vi "_emi_New Named Loop Deprecated.vi"(2 "Loop Enabled(T)":bool=TRUE, 7 "Loop Name(\"\")":string, 9 "error in (no error)":errorcluster) -> (6 "Loop ID":u16, 10 "error out":errorcluster)   [LabVIEW 2010]
doc: "Create a new loop vased on name. NOT IMPLEMENTED"
uses:
  _emi_Loop control int action.ctl
  emi_Set Status Loop.vi
  _emi_GFV Loop Running.vi
  _emi_GFV Loop Enable.vi
  _emi_GFV Loop Linking.vi
  _emi_GFV stop a loop so it can reset.vi
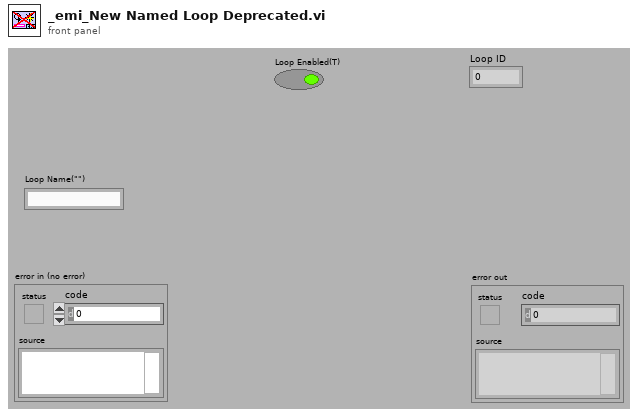
[diagram p1: front panel]
types:
  T1 = typedef "_emi_Loop control int action.ctl" = enum16{"Init index", "Get index", "Set index", "Get Size"}
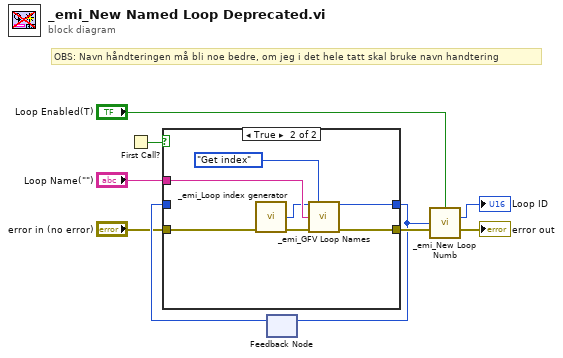
[diagram p0: block diagram]
diagram:
  # "OBS: Navn håndteringen må bli noe bedre, om jeg i det hele tatt skal bruke navn handtering"
  n1 = First Call?() -> (First Call?: T/F=w9:bool)
  n2 = feedback #1() -> (w7:u16)  [unwired: 1 in]
  n3 = case shown="True" w9 {
    tunnel: "Loop Name(\"\")" -> [_ w15]
    tunnel: [w11 w14] -> w3
    tunnel: w7 -> [w11 _]
    tunnel: "error in (no error)" -> [w10 w18]
    tunnel: [w10 w16] -> w5
    frame False {
    }
    frame True {
      n4 = call "_emi_Loop index generator.vi"("error in (no error)"=w18) -> ("Loop ID out"=w12:u16, "error out"=w17:errorcluster)  [unwired: 13 in]
      n5 = call "_emi_GFV Loop Names.vi"("Loop Index/Numb"=w12, "Action(Get Index)"=_emi_Loop_control_int_action."Get index", "Loop Name(\"\")"=w15, "error in (no error)"=w17) -> ("Index out"=w14:u16, "error out"=w16:errorcluster)  [unwired: 8 in, 2 out]
    }
  }
  n6 = feedback-in #1(w3) -> ()
  n7 = call "_emi_New Loop Numb.vi"("Loop Enable (T)"="Loop Enabled(T)", "Loop Index"=w3, "error in (no error)"=w5) -> ("Loop ID"=→"Loop ID":u16, "error out"=→"error out":errorcluster)  [unwired: 11 in]
